vi "Alarms Clear.vi"(7 "Clear Alarms In":bool=TRUE, 8 "Error In":errorcluster, 11 "Alarms Data In":T1) -> (0 "Error Out":errorcluster, 3 "Alarms Data Out":T1)   [LabVIEW 2014]
uses:
  Controls/Alarms Data.ctl
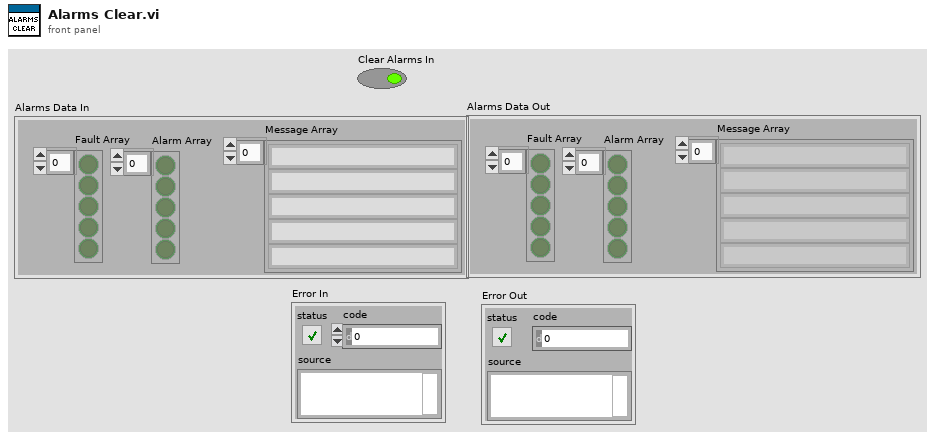
[diagram p1: front panel]
types:
  T1 = typedef "Alarms Data.ctl" = cluster{"Message Array":string[], "Fault Array":bool[], "Alarm Array":bool[]}
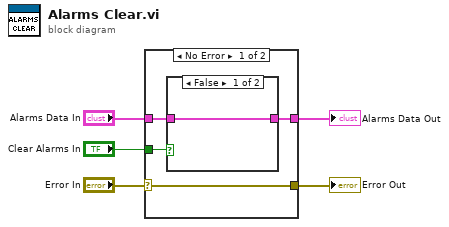
[diagram p0: block diagram]
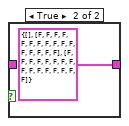
[diagram p2: hidden frame]
diagram:
  n1 = case shown="No Error" "Error In" {
    selector: "Error In" -> [w9 w13]
    tunnel: [w9 w13] -> w4
    tunnel: "Alarms Data In" -> [w7 w12]
    tunnel: [w6 w12] -> w2
    tunnel: "Clear Alarms In" -> [w8 _]
    frame No Error {
      n2 = case shown="False" w8 {
        tunnel: w7 -> [w10 _]
        tunnel: [w10 T1 {"Message Array"=[], "Fault Array"=[FALSE, FALSE, FALSE, FALSE, FALSE, FALSE, FALSE, FALSE, FALSE, FALSE, FALSE, FALSE, FALSE, FALSE, FALSE, FALSE], "Alarm Array"=[FALSE, FALSE, FALSE, FALSE, FALSE, FALSE, FALSE, FALSE, FALSE, FALSE, FALSE, FALSE, FALSE, FALSE, FALSE, FALSE]} ("Alarms Data In")] -> w6
        frame False {
        }
        frame True {
        }
      }
    }
    frame Error {
    }
  }
  "Error Out" <- w4
  "Alarms Data Out" <- w2
